vi "LookUpTable Entry.vi"(7 "Type":T1=enum."Input/Read", 8 "error in":errorcluster, 9 "Name":string, 10 "LUT":variant) -> (0 "error out":errorcluster, 2 "LUT":variant)   [LabVIEW 2026, in "SystemMonitor Deployment Hooks.lvlib"]
uses:
  SystemMonitor Deployment Hooks.lvlib
  Types/Channel Mode.ctl
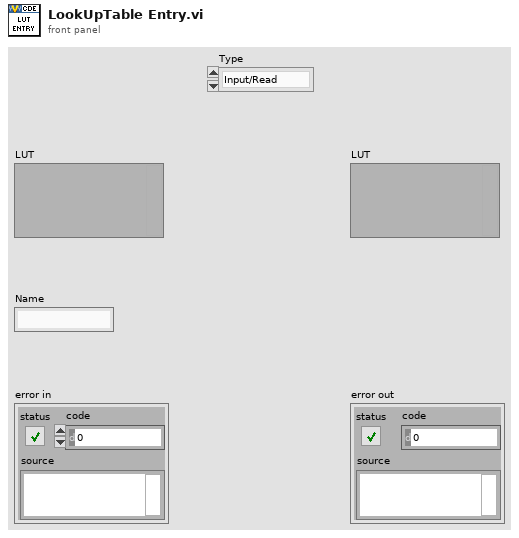
[diagram p1: front panel]
types:
  T1 = typedef "SystemMonitor Deployment Hooks.lvlib/Channel Mode.ctl" = enum16{"Output/Write", "Input/Read", "Input/ReadWrite"}
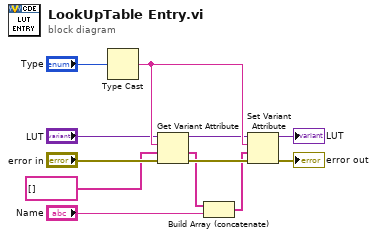
[diagram p0: block diagram]
diagram:
  n1 = Type Cast(x="Type") -> (*(type *) &x=w5:string)  [unwired: 1 in]
  n2 = Get Variant Attribute(Variant="LUT", name=w5, default value (empty Variant)=string[] [], error in="error in") -> (duplicate Variant=w3:variant, value=w7:string[], error out=w10:errorcluster)  [unwired: 1 out]
  n3 = Build Array (concatenate)(w7, "Name") -> (w8:string[])
  n4 = Set Variant Attribute(Variant=w3, name=w5, value=w8, error in=w10) -> (Variant out=→"LUT":variant, error out=→"error out":errorcluster)  [unwired: 1 out]
